vi "SRV_Queue_Dequeue Element.vi"(6 "timeout in ms (-1)":i32=-1, 8 "error in (no error)":errorcluster, 11 "Command-Data Queue":refnum<queue>) -> (0 "error out":errorcluster, 1 "Data":variant, 2 "Command":string, 3 "Command-Data Queue out":refnum<queue>, 4 "timed out?":bool, 5 "Command History":string[](array[string]))   [LabVIEW 2014]
doc: "Dequeues an element from the referenced Command-Data Queue.\n\n\nAuthor: Mike Schultz - Logic PD"
uses:
  SRV_Command-Data Queue Data Type.ctl
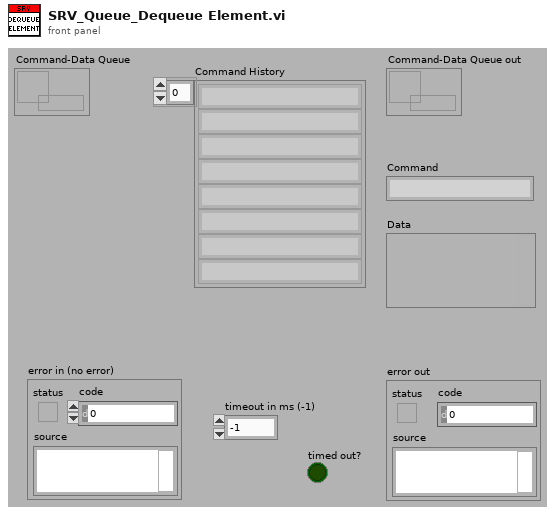
[diagram p1: front panel]
types:
  T1 = typedef "SRV_Command-Data Queue Data Type.ctl" = cluster{"Command":string, "Data":variant}
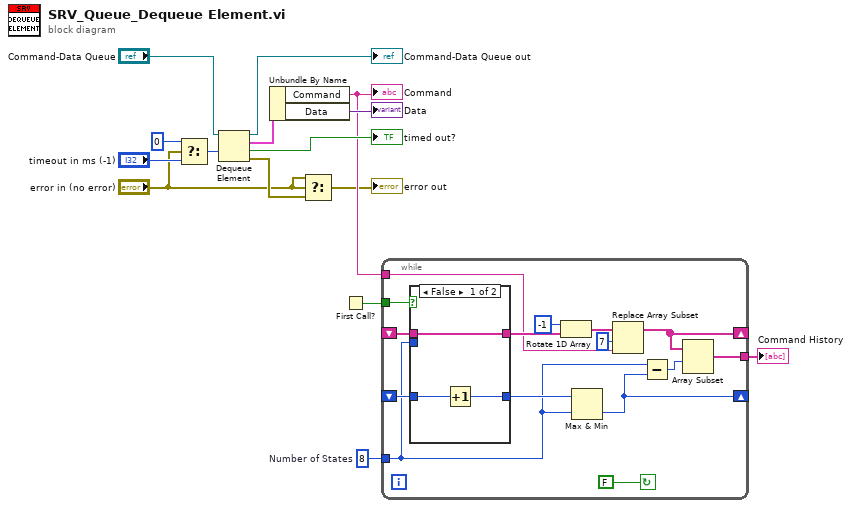
[diagram p0: block diagram]
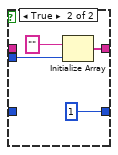
[diagram p2: hidden frame]
diagram:
  w9 = 8  # Number of States
  n1 = Select(t=0, s="error in (no error)", f="timeout in ms (-1)") -> (s? t:f=w3:i32)
  n2 = Dequeue Element(queue="Command-Data Queue", timeout in ms (-1)=w3) -> (queue out=→"Command-Data Queue out":refnum<queue>, element=w12:T1, timed out?=→"timed out?":bool, error out=w6:errorcluster)  [unwired: 1 in]
  n3 = Unbundle By Name(w12) -> ("Command"=w7:string, "Data"=→"Data":variant)
  "Command" <- w7
  n4 = Select(t="error in (no error)", s="error in (no error)", f=w6) -> (s? t:f=→"error out":errorcluster)
  n5 = First Call?() -> (First Call?: T/F=w8:bool)
  n6 = while {
    shift-right: [w20] -> _
    shift-left: _ -> [w30]
    shift-right: [w16] -> _
    shift-left: _ -> [w29]
    tunnel: w8 -> [w28]
    tunnel: w9 -> [w17]
    tunnel: w7 -> [w22]
    tunnel: [w19] -> w10
    stop <- FALSE continue-if-true
    n7 = case shown="False" w28 {
      tunnel: [w33 w36] -> w23
      tunnel: w30 -> [w33 _]
      tunnel: w29 -> [w32 _]
      tunnel: [w31 1] -> w27
      tunnel: w17 -> [_ w34]
      frame False {
        n8 = Increment(x=w32) -> (x+1=w31:i32)
      }
      frame True {
        n9 = Initialize Array("", w34) -> (w36:string[])
      }
    }
    n10 = Rotate 1D Array(1:w23, 2:-1 ("n")) -> (0:w24:string[])
    n11 = Max & Min(x=w27, y=w17) -> (min(x,y)=w16:i32)  [unwired: 1 out]
    n12 = Replace Array Subset(array=w24, new element=w22, index=7) -> (w20:string[])
    n13 = Subtract(x=w17, y=w16) -> (x-y=w18:i32)
    n14 = Array Subset(array=w20, index=w18) -> (w19:string[])  [unwired: 1 in]
  }
  "Command History" <- w10
